vi "GL_DRCchannel.vi"() -> ()   [LabVIEW 2019]
panel:
  in  "CHANNEL":bool
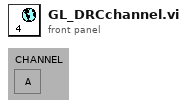
[diagram p1: front panel]
diagram:
